vi "_db.vi"(7 "command":T1, 8 "error in (no error)":errorcluster, 9 "Message VI Option":i32=8 format="%x", 10 "ui_bar":refnum<class "UI_ProgressDlg.lvclass">, 11 "name":string) -> (0 "error out":errorcluster, 1 "created new?":bool, 3 "ui_bar out":refnum<class "UI_ProgressDlg.lvclass">)   [LabVIEW 2014]
uses:
  <userlib>/NEVSTOP_ProgressDlg/MSGFramework(dev).lvclass
  <vilib>/Utility/notifier.llb/Notifier SRdB command.ctl
  <userlib>/NEVSTOP_ProgressDlg/UI_ProgressDlg.lvclass
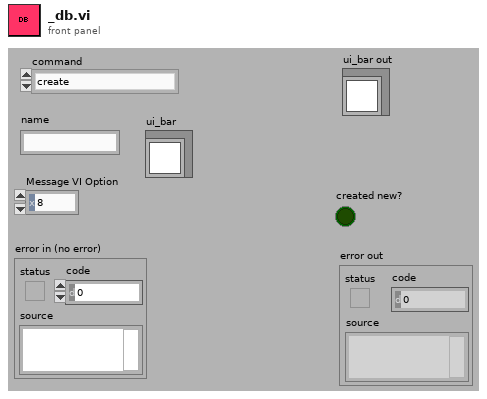
[diagram p1: front panel]
types:
  T1 = typedef "Notifier SRdB command.ctl" = enum16{"create", "destroy", "cleanUp"}
  T2 = cluster{"db":refnum<class "MSGFramework(dev).lvclass">, "Count":i32}[]
  T3 = cluster{"db":refnum<class "MSGFramework(dev).lvclass">, "Count":i32}
  T4 = cluster{"MSGFramwork out":refnum<class "MSGFramework(dev).lvclass">, i32}
  T5 = cluster{"MSGFramwork out":refnum<class "MSGFramework(dev).lvclass">, i32}[]
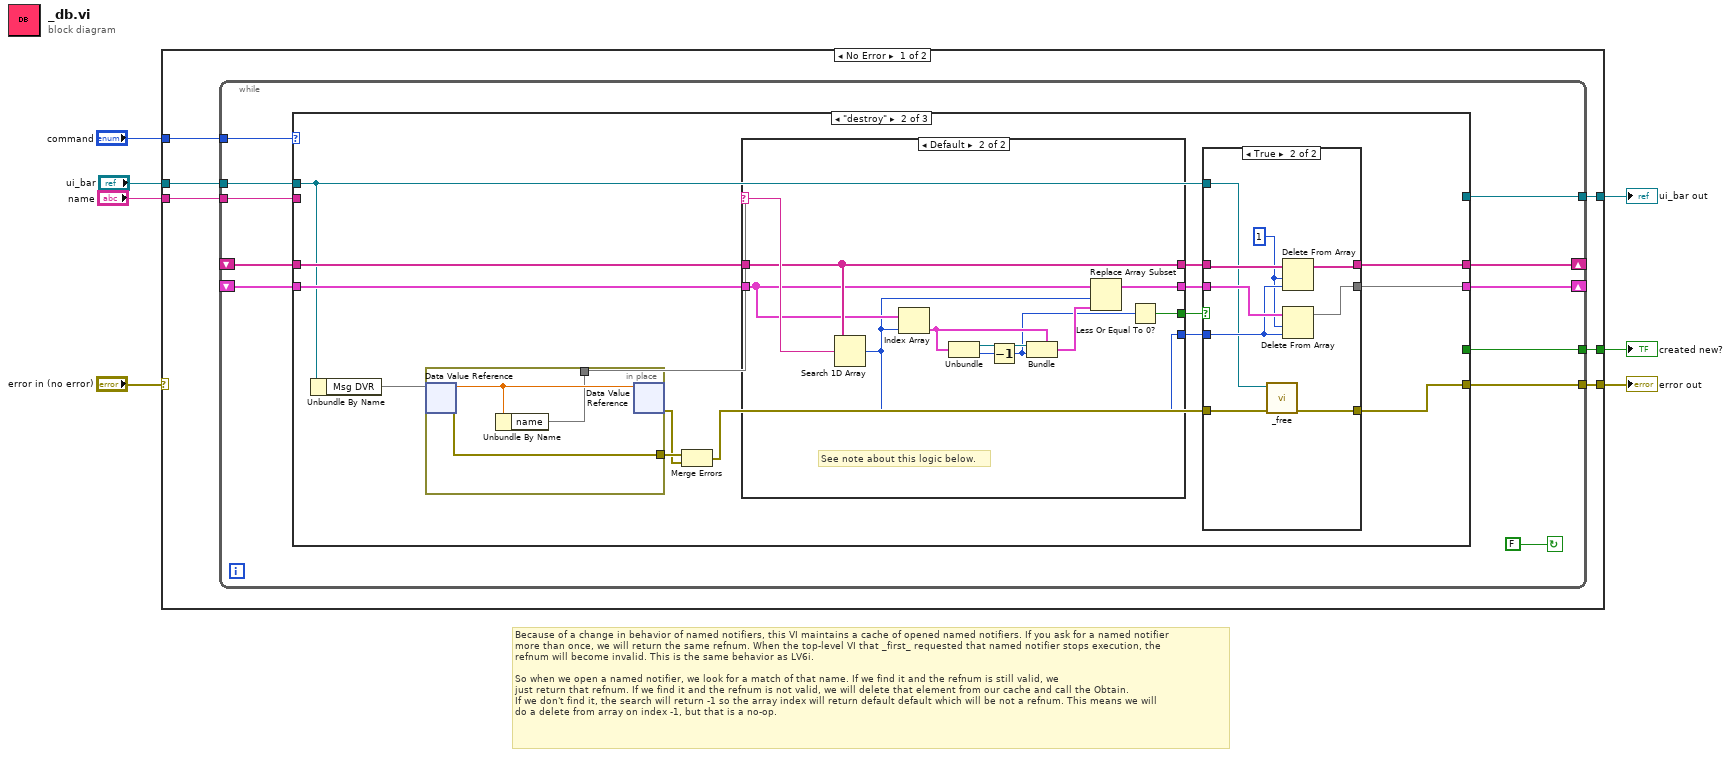
[diagram p0: block diagram]
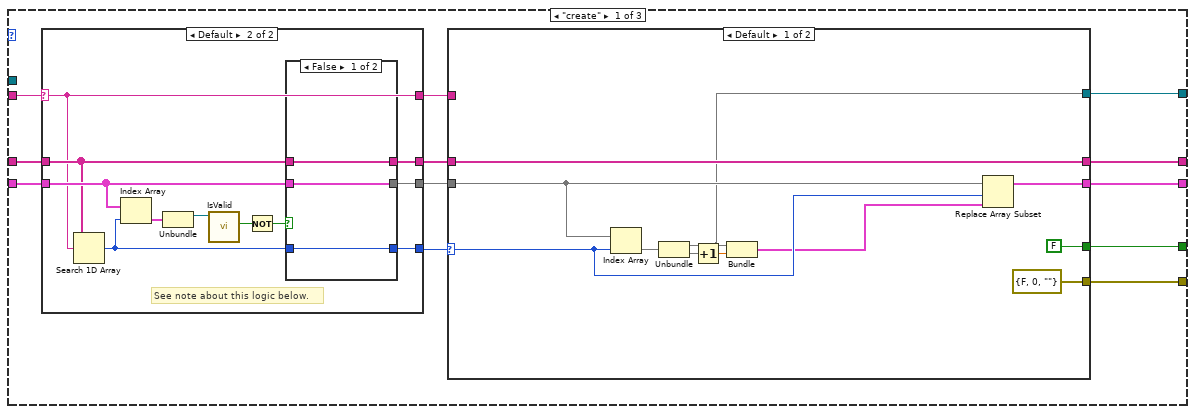
[diagram p2: hidden frame]
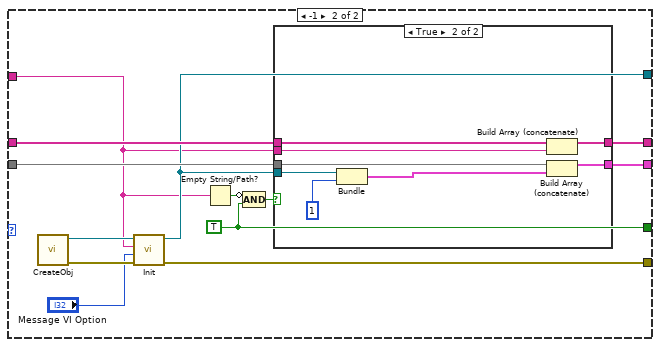
[diagram p3: hidden frame]
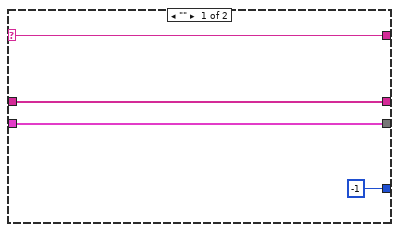
[diagram p5: hidden frame]
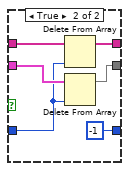
[diagram p6: hidden frame]
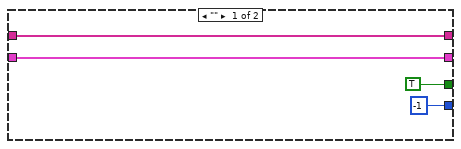
[diagram p8: hidden frame]
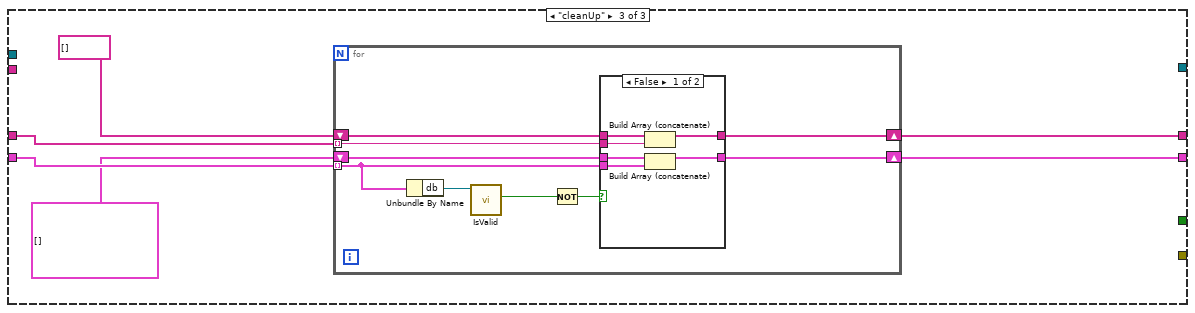
[diagram p9: hidden frame]
diagram:
  # "Because of a change in behavior of named notifiers, this VI maintains a cache of opened named notifiers. If you ask for a named notifier\nmore than once, we will return the same refnum. When the top-level VI that _first_ requested that named notifier stops execution, the\nrefnum will become invalid. This is the same behavior as LV6i.\n\nSo when we open a named notifier, we look for a match of that name. If we find it and the refnum is still valid, we\njust return that refnum. If we find it and the refnum is not valid, we will delete that element from our cache and call the Obtain.\nIf we don't find it, the search will return -1 so the array index will return default default which will be not a refnum. This means we will\ndo a delete from array on index -1, but that is a no-op."
  n1 = case shown="No Error" "error in (no error)" {
    selector: "error in (no error)" -> [_ w164]
    tunnel: [w13 w164] -> w3
    tunnel: [w12 FALSE ("created new?")] -> w2
    tunnel: [w11 _] -> w7
    tunnel: "name" -> [w10 _]
    tunnel: "command" -> [w9 _]
    tunnel: "ui_bar" -> [w8 _]
    frame No Error {
      n2 = while {
        shift-right: [w18] -> _
        shift-left: _ -> [w24]
        shift-right: [w19] -> _
        shift-left: _ -> [w23]
        tunnel: [w22] -> w11
        tunnel: [w21] -> w13
        tunnel: [w20] -> w12
        tunnel: w10 -> [w16]
        tunnel: w9 -> [w15]
        tunnel: w8 -> [w14]
        stop <- FALSE continue-if-true
        n3 = case shown="\"destroy\"" w15 {
          tunnel: w24 -> [w35 w109 w142]
          tunnel: w23 -> [w34 w108 w143]
          tunnel: [w33 _ _] -> w22
          tunnel: [w32 w102 _] -> w21
          tunnel: [w31 _ _] -> w20
          tunnel: [w28 w98 w144] -> w19
          tunnel: [w27 w100 w145] -> w18
          tunnel: w16 -> [w25 _ _]
          tunnel: w14 -> [_ w95 _]
          frame "create" {
            n4 = case shown="Default" w25 {
              selector: w25 -> [w74 w79]
              tunnel: [w74 w79] -> w36
              tunnel: w35 -> [w73 w80]
              tunnel: w34 -> [w71 w85]
              tunnel: [w73 w84] -> w26
              tunnel: [w71 w83] -> w29
              tunnel: [-1 ("index") w82] -> w30
              frame "" {
              }
              frame Default {
                # "See note about this logic below."
                n5 = Search 1D Array(1D array=w80, element=w79) -> (index of element=w78:i32)  [unwired: 1 in]
                n6 = Index Array(array=w85, index=w78) -> (element=w77:T3)
                n7 = Unbundle(w77) -> ("db"=w75:refnum<class "MSGFramework(dev).lvclass">)  [unwired: 1 out]
                n8 = call <userlib>:"IsValid.vi"("MSGFramwork in"=w75) -> ("valid?"=w81:bool)  [unwired: 8 in, 2 out]
                n9 = Not(x=w81) -> (.not. x?=w76:bool)
                n10 = case shown="False" w76 {
                  tunnel: w78 -> [w86 w89]
                  tunnel: w85 -> [w88 w94]
                  tunnel: w80 -> [w87 w93]
                  tunnel: [w87 w92] -> w84
                  tunnel: [w88 w91] -> w83
                  tunnel: [w86 -1 ("index of element")] -> w82
                  frame False {
                  }
                  frame True {
                    n11 = Delete From Array(array=w93, index=w89) -> (array with subset deleted=w92:string[])  [unwired: 1 in, 1 out]
                    n12 = Delete From Array(array=w94, index=w89) -> (array with subset deleted=w91)  [unwired: 1 in, 1 out]
                  }
                }
              }
            }
            n13 = case shown="Default" w30 {
              selector: w30 -> [w41 _]
              tunnel: w36 -> [_ w49]
              tunnel: [w40 w51] -> w33
              tunnel: [errorcluster {"status"=FALSE, "code"=0, "source"=""} ("error out") w60] -> w32
              tunnel: [FALSE ("created new?") w50] -> w31
              tunnel: w29 -> [w43 w56]
              tunnel: [w42 w57] -> w28
              tunnel: [w47 w58] -> w27
              tunnel: w26 -> [w47 w59]
              frame Default {
                n14 = Index Array(array=w43, index=w41) -> (element=w44)
                n15 = Unbundle(w44) -> (w40, w39)
                n16 = Increment(x=w39) -> (x+1=w37:dbl)
                n17 = Bundle(w40, w37) -> (w38:cluster{void, dbl})  [unwired: 1 in]
                n18 = Replace Array Subset(array=w43, new element=w38, index=w41) -> (w42:cluster{void, dbl}[])
              }
              frame -1 {
                w50 = TRUE ("created new?")
                n19 = call <userlib>:"CreateObj.vi"() -> ("error out"=w53:errorcluster, "MSGFramwork out"=w52:refnum<class "MSGFramework(dev).lvclass">)  [unwired: 10 in]
                n20 = call <userlib>:"Init.vi"("error in (no error)"=w53, "Message VI Option"="Message VI Option", "name(\"\" as default)"=w49, "MSGFramwork in"=w52) -> ("error out"=w60:errorcluster, "MSGFramwork out"=w51:refnum<class "MSGFramework(dev).lvclass">)  [unwired: 6 in]
                n21 = Empty String/Path?(string/path=w49) -> (empty?=w55:bool)
                n22 = Compound Arithmetic op=AND(invert w55, w50) -> (w54:bool)
                n23 = case shown="True" w54 {
                  tunnel: w59 -> [w62 w70]
                  tunnel: [w62 w68] -> w58
                  tunnel: [w61 w67] -> w57
                  tunnel: w56 -> [w61 w69]
                  tunnel: w51 -> [_ w64]
                  tunnel: w49 -> [_ w66]
                  frame False {
                  }
                  frame True {
                    n24 = Bundle("MSGFramwork out"=w64, 1) -> (w65:T4)  [unwired: 1 in]
                    n25 = Build Array (concatenate)(w70, w66) -> (w68:string[])
                    n26 = Build Array (concatenate)(w69, w65) -> (w67:T5)
                  }
                }
              }
            }
          }
          frame "destroy" {
            n27 = Unbundle By Name(w95) -> ("Msg DVR"=w107)
            n28 = in-place {
              in-place-border: [w123] -> w106
              in-place-border: [w122] -> w104
              n29 = in-place-dvr #1(w107) -> (w124:dbl, w123:errorcluster)
              n30 = Unbundle By Name(w124) -> ("name"=w122)
              n31 = in-place-dvr #1(w124) -> (w105:errorcluster)  [unwired: 1 out]
            }
            n32 = Merge Errors(w106, w105) -> (w103:errorcluster)
            n33 = case shown="Default" w104 {
              selector: w104 -> [_ w139]
              tunnel: w109 -> [w128 w135]
              tunnel: w108 -> [w127 w134]
              tunnel: [w128 w135] -> w99
              tunnel: [w127 w133] -> w97
              tunnel: [TRUE w131] -> w101
              tunnel: [-1 ("index of element") w129] -> w96
              frame "" {
              }
              frame Default {
                # "See note about this logic below."
                n34 = Search 1D Array(1D array=w135, element=w139) -> (index of element=w129:i32)  [unwired: 1 in]
                n35 = Index Array(array=w134, index=w129) -> (element=w138:T3)
                n36 = Unbundle(w138) -> ("db"=w137:refnum<class "MSGFramework(dev).lvclass">, "Count"=w136:i32)
                n37 = Decrement(x=w136) -> (x-1=w130:i32)
                n38 = Bundle(cluster=w138, "db"=w137, "Count"=w130) -> (w132:T3)
                n39 = Replace Array Subset(array=w134, new element=w132, index=w129) -> (w133:T2)
                n40 = Less Or Equal To 0?(x=w130) -> (x <= 0?=w131:bool)
              }
            }
            n41 = case shown="True" w101 {
              tunnel: w103 -> [w112 w114]
              tunnel: w95 -> [_ w115]
              tunnel: [w112 w113] -> w102
              tunnel: [w111 w120] -> w100
              tunnel: w99 -> [w111 w121]
              tunnel: [w110 w118] -> w98
              tunnel: w97 -> [w110 w119]
              tunnel: w96 -> [_ w117]
              frame False {
              }
              frame True {
                w116 = 1 ("length")
                n42 = call <userlib>:"_free.vi"("error in (no error)"=w114, "MSGFramwork in"=w115) -> ("error out"=w113:errorcluster)  [unwired: 8 in, 1 out]
                n43 = Delete From Array(array=w121, length=w116, index=w117) -> (array with subset deleted=w120:string[])  [unwired: 1 out]
                n44 = Delete From Array(array=w119, length=w116, index=w117) -> (array with subset deleted=w118)  [unwired: 1 out]
              }
            }
          }
          frame "cleanUp" {
            n45 = for {
              shift-right: [w153] -> w145
              shift-left: string[] [] -> [w154]
              tunnel: w143 -> [w148] mode=indexing
              shift-right: [w152] -> w144
              shift-left: T2 [] -> [w150]
              tunnel: w142 -> [w151] mode=indexing
              n46 = Unbundle By Name(w148) -> ("db"=w146:refnum<class "MSGFramework(dev).lvclass">)
              n47 = call <userlib>:"IsValid.vi"("MSGFramwork in"=w146) -> ("valid?"=w149:bool)  [unwired: 8 in, 2 out]
              n48 = Not(x=w149) -> (.not. x?=w147:bool)
              n49 = case shown="False" w147 {
                tunnel: w154 -> [w160 w162]
                tunnel: w148 -> [w156 _]
                tunnel: [w159 w162] -> w153
                tunnel: [w157 w161] -> w152
                tunnel: w151 -> [w158 _]
                tunnel: w150 -> [w155 w161]
                frame False {
                  n50 = Build Array (concatenate)(w160, w158) -> (w159:string[])
                  n51 = Build Array (concatenate)(w155, w156) -> (w157:T2)
                }
                frame True {
                }
              }
            }
          }
        }
      }
    }
    frame Error {
      (unwired) refnum<k0> refnum
    }
  }
  "created new?" <- w2
  "error out" <- w3
  "ui_bar out" <- w7
